vi "Special Cases for Incoming Data.vi"(8 "error in (no error)":errorcluster, 11 "Data In":string) -> (0 "error out":errorcluster, 1 "After Special Case":string, 2 "Special Case":string, 3 "Data Out":string, 5 "Before Special Case":string)   [LabVIEW 2018]
uses:
  controls/Special Cases from XPert.ctl
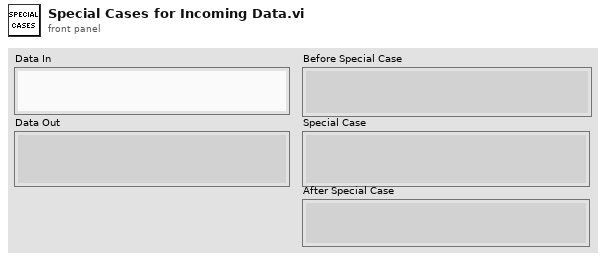
[diagram p1: front panel]
types:
  T1 = typedef "Special Cases from XPert.ctl" = string
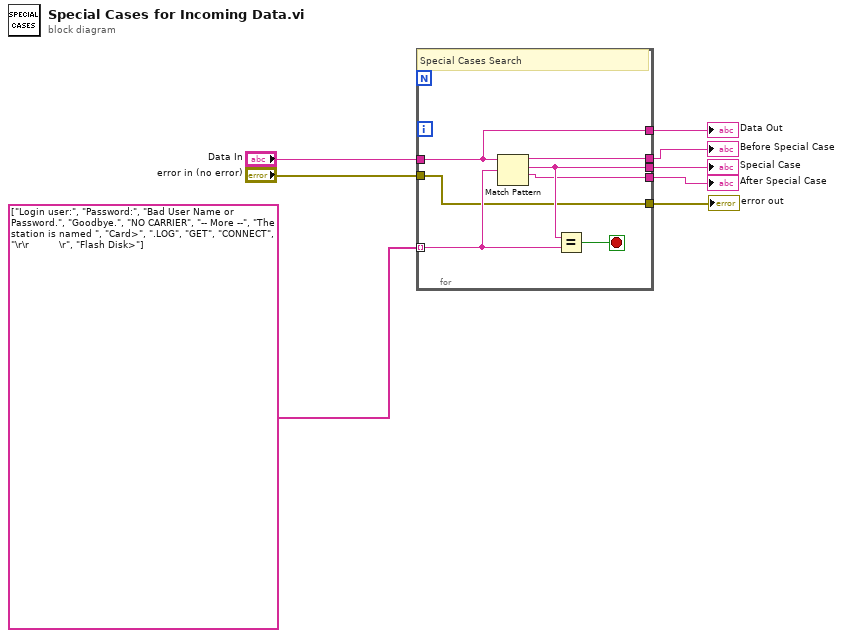
[diagram p0: block diagram]
diagram:
  n1 = for {
    tunnel: "Data In" -> [w12]
    tunnel: T1[] ["Login user:", "Password:", "Bad User Name or Password.", "Goodbye.", "NO CARRIER", "-- More --", "The station is named ", "Card>", ".LOG", "GET", "CONNECT", "\r\r          \r", "Flash Disk>"] -> [w14] mode=indexing
    tunnel: [w13] -> w1
    tunnel: [w12] -> w7
    tunnel: "error in (no error)" -> [w11]
    tunnel: [w11] -> w6
    tunnel: [w10] -> w3
    tunnel: [w9] -> w2
    stop <- w15 stop-if-true
    # "Special Cases Search"
    n2 = Match Pattern(string=w12, regular expression=w14) -> (before substring=w9:string, match substring=w13:string, after substring=w10:string)  [unwired: 1 in, 1 out]
    n3 = Equal?(x=w13, y=w14) -> (x = y?=w15:bool)
  }
  "Data Out" <- w7
  "error out" <- w6
  "Special Case" <- w1
  "Before Special Case" <- w2
  "After Special Case" <- w3
